vi "2_AdvancedDemo_TH260Histo.vi"() -> ()   [LabVIEW 2017]
uses:
  Types/TH260_InputChannel.ctl
  Types/TH260_UIThread_Cmds.ctl
  Types/TH260_UIThread_Data.ctl
  _lib/PQ/TimeHarp260/TH260_InitInfo.ctl
  _lib/PQ/TimeHarp260/TH260_MeasMode.ctl
  _lib/PQ/TimeHarp260/TH260_TimingMode.ctl
  <vilib>/Utility/error.llb/DialogType.ctl
  _lib/PQ/TimeHarp260/th260lib_x86_x64_UIThread.llb/TH260_DllPath_global.vi
  <vilib>/Utility/error.llb/Error Cluster From Error Code.vi
  _lib/PQ/TimeHarp260/TH260_LibVersion_global.vi
  <vilib>/ErrorRing/Error Ring.xnode
panel:
  in  "Settings":bool=TRUE
  in  "Run continuously":bool=TRUE caption="Conti."
  in  "Start":bool
  in  "Scale":bool
  out "CountRates":i32[](graph)
  in  "HistoLength":i32(ring)=6 caption="Num Bins" items=["1024", "2048", "4096", "8192", "16384", "32768"]
  in  "OvlLevel":u32=100000 caption="Ovl.Level" min=1 step=1
  in  "StopOvl.":bool=TRUE
  in  "AcqTime":i32=1000 caption="Acqu.     ms" min=1 max=360000000 step=1
  in  "Binning":i32(ring) caption="Resol.      ps" items=["25", "50", "100", "200", "400", "800", "1600", "3200", "6400", "12800", "25600", "51200", "102400", "204800", "409600", "819200", "1638400", "3276800", "6553600", "13107200", "26214400", "52428800"]
  in  "HistoOffset":i32 caption="Offset      ns" min=0 max=100000000 step=1
  out "HistoGraph":T1(graph)={0.0, "Resolution"=0.001, "Histogram"=array8x1024[8192 elements]}
  in  "SyncTrgEdge":i32(ring) caption="Edge" items=["falling", "rising"]
  in  "SyncTrgLevel":i32=-100 caption="Level        mV" min=-1200 max=1200 step=1
  in  "SyncCFDLevel":i32=-100 caption="Level        mV" min=-1200 max=0 step=1
  in  "SyncZeroX":i32=-10 caption="ZeroCr.    mV" min=-40 max=0 step=1
  in  "SyncDivider":i32(ring)=3 caption="Divider" items=["1", "2", "4", "8"]
  in  "SyncOffset":i32 caption="Offset        ps" min=-99999 max=99999 step=1
  in  "Channels":T2[](array[typedef])=[{"Name"="Inp.Chan 1", "Enable"=TRUE, "Offset"=0, "CFDLevel"=50, "ZeroX"=10, "dtcode"=0, "TrgLevel"=-100, "TrgEdge"=0}, {"Name"="Inp.Chan 2", "Enable"=TRUE, "Offset"=0, "CFDLevel"=50, "ZeroX"=10, "dtcode"=0, "TrgLevel"=-100, "TrgEdge"=0}, {"Name"="Inp.Chan 3", "Enable"=TRUE, "Offset"=0, "CFDLevel"=50, "ZeroX"=10, "dtcode"=0, "TrgLevel"=-100, "TrgEdge"=0}, {"Name"="Inp.Chan 4", "Enable"=TRUE, "Offset"=0, "CFDLevel"=50, "ZeroX"=10, "dtcode"=0, "TrgLevel"=-100, "TrgEdge"=0}, {"Name"="Inp.Chan 5", "Enable"=TRUE, "Offset"=0, "CFDLevel"=50, "ZeroX"=10, "dtcode"=0, "TrgLevel"=-100, "TrgEdge"=0}, {"Name"="Inp.Chan 6", "Enable"=TRUE, "Offset"=0, "CFDLevel"=50, "ZeroX"=10, "dtcode"=0, "TrgLevel"=-100, "TrgEdge"=0}, {"Name"="Inp.Chan 7", "Enable"=TRUE, "Offset"=0, "CFDLevel"=50, "ZeroX"=10, "dtcode"=0, "TrgLevel"=-100, "TrgEdge"=0}, {"Name"="Inp.Chan 8", "Enable"=TRUE, "Offset"=0, "CFDLevel"=50, "ZeroX"=10, "dtcode"=0, "TrgLevel"=-100, "TrgEdge"=0}] {"TrgEdge" items=["falling", "rising"]; "TrgLevel" min=-1200 max=1200 step=1; "dtcode" items=["24", "44", "66", "88", "112", "135", "160", "180"]; "ZeroX" min=-40 max=0 step=1; "Offset" min=-99999 max=99999 step=1; "CFDLevel" min=-1200 max=0 step=1}
  out "SyncRate":string="Sync Rate: 0 cps\n"
  out "OverFlow":bool caption="Overflow:"
  out "Status":string="Initialized!"
  # "Histogram"
  # "Sync"
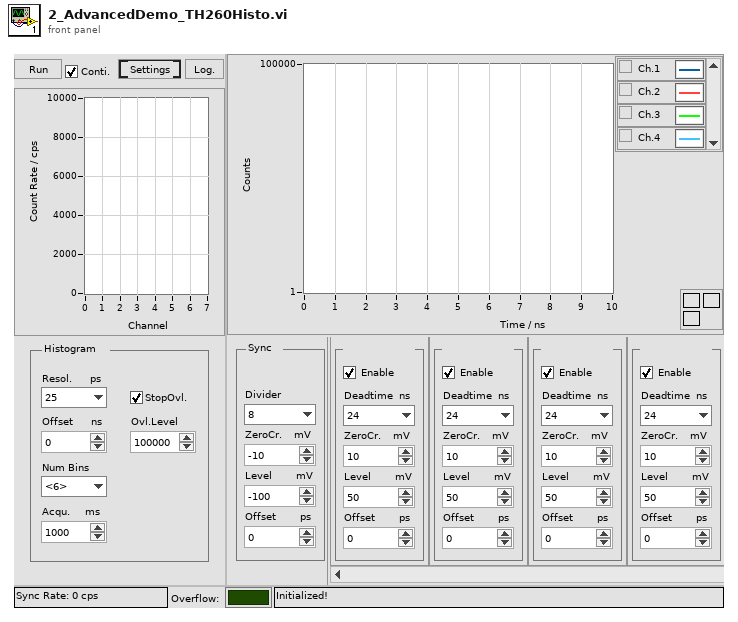
[diagram p1: front panel]
types:
  T1 = cluster{dbl, "Resolution":dbl, "Histogram":u32[][]}
  T2 = typedef "TH260_InputChannel.ctl" = cluster{"Name":string, "Enable":bool, "Offset":i32, "CFDLevel":i32, "ZeroX":i32, "dtcode":i32, "TrgLevel":i32, "TrgEdge":i32}
  T3 = typedef "TH260_UIThread_Data.ctl" = cluster{"Init Info":T4, "DevIdx":i32, "Channels":T2[], "CurrentChannels":i32[], "AcqTime":i32, "Binning":i32, "HistoOffset":i32, "HistoLen":i32, "StopOvl.":bool, "OvlLevel":u32, "StartMeas":bool, "HistoLength":i32, "Resolution":dbl, "Run cont.":bool, "Status":string, "SyncRate":i32, "BitShift":i32, "HistoAcqTime":dbl, "SyncTrgEdge":i32, "SyncTrgLevel":i32, "SyncCFDLevel":i32, "SyncZeroX":i32, "SyncDivider":i32, "SyncOffset":i32}
  T4 = typedef "TH260_InitInfo.ctl" = cluster{"Library Version":string, "Serial No.":string, "Model":string, "Partnum":string, "Version":string, "features":i32, "nchannels":i32, "Base Resolution":dbl, "Bin Steps":i32}
  T5 = typedef "TH260_UIThread_Cmds.ctl" = enum16{"Idle", "Init", "SetInpChanEnable", "SetInpChanOffset", "SetInpChanCFD", "SetInpChanTrg", "SetInpChanDeadtime", "SetSyncDivider", "SetSyncCFD", "SetSyncTrg", "SetSyncOffset", "SetBinning", "SetHistoOffset", "SetHistoLen", "SetStopOvl", "SetBitShift", "SetHistoAcqTime", "GetRates", "StartMeas", "StopMeas", "AbortMeas", "GetResolution", "GetHisto", "ReadFiFo", "WriteStatus", "Resize", "EnableControls", "DisableControls", "Error", "Exit"}
  T6 = enum8{"Enabled", "Disabled", "Disabled and Grayed Out"}
  T7 = typedef "TH260_TimingMode.ctl" = i32
  T8 = typedef "TH260_MeasMode.ctl" = i32
  T9 = typedef "DialogType.ctl" = u16
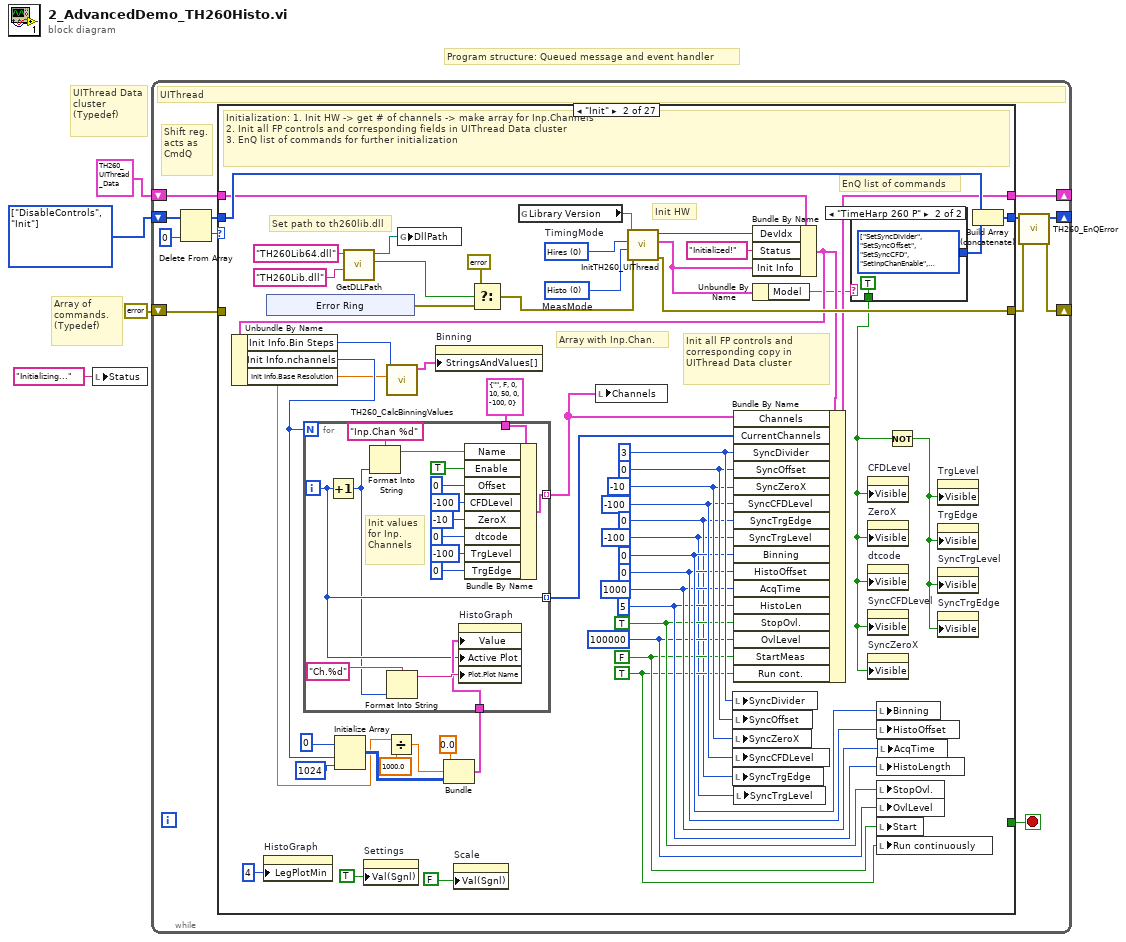
[diagram p0: block diagram]
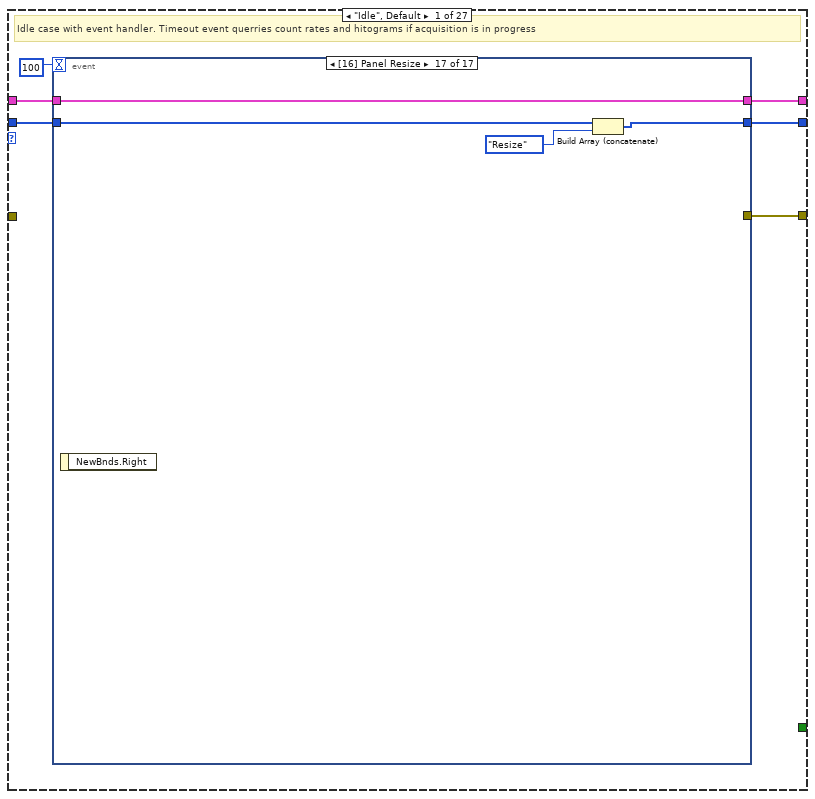
[diagram p2: hidden frame]
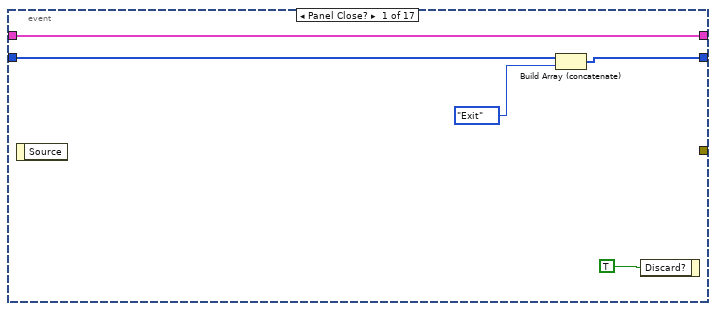
[diagram p3: hidden frame]
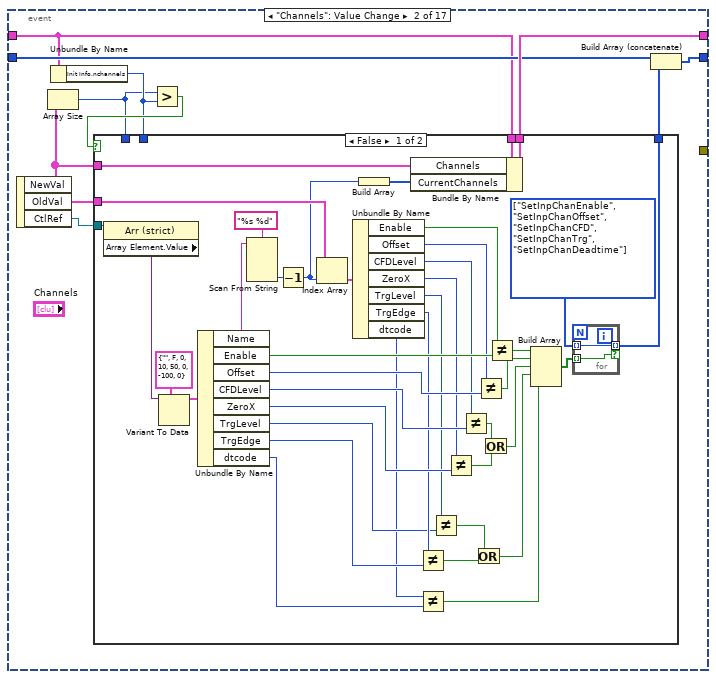
[diagram p4: hidden frame]
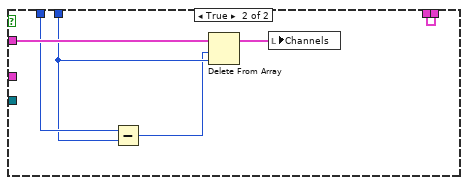
[diagram p5: hidden frame]
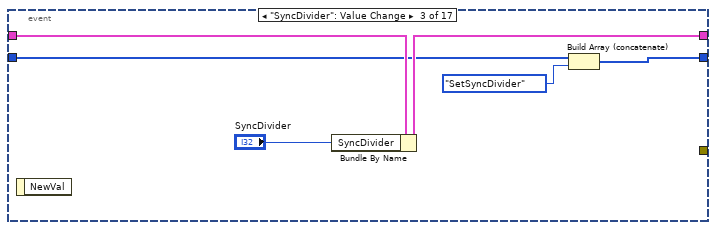
[diagram p6: hidden frame]
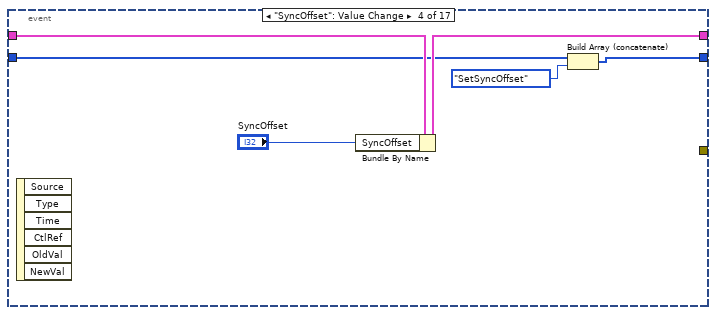
[diagram p7: hidden frame]
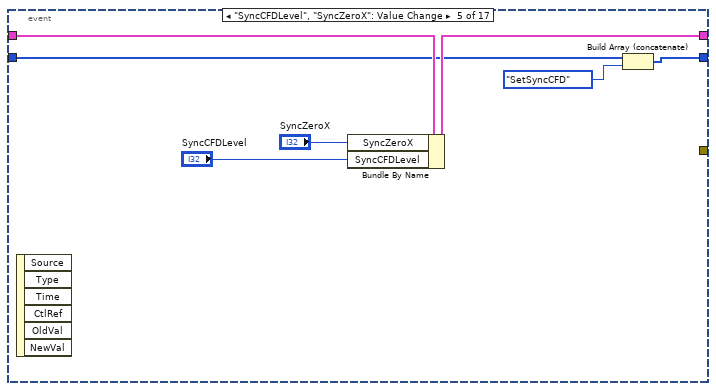
[diagram p8: hidden frame]
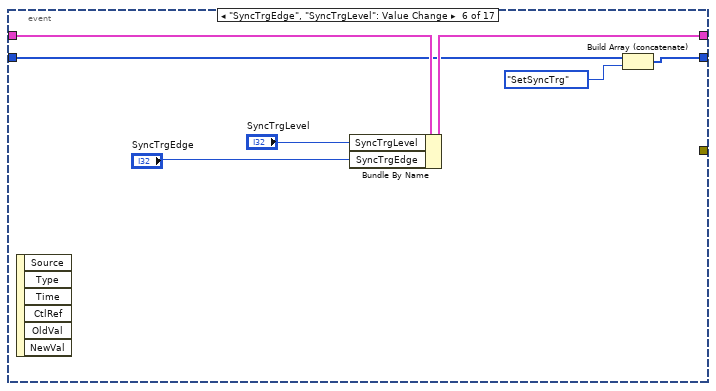
[diagram p9: hidden frame]
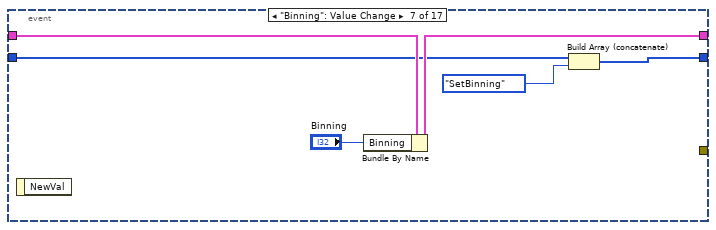
[diagram p10: hidden frame]
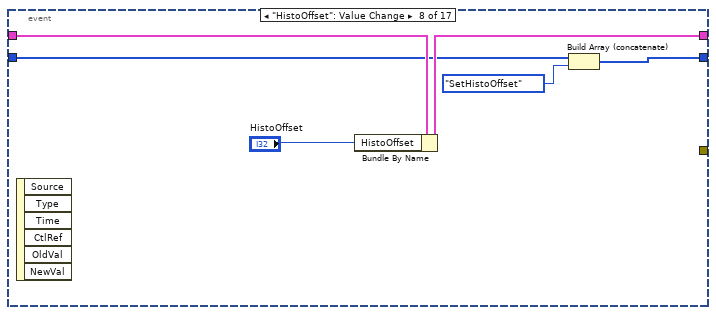
[diagram p11: hidden frame]
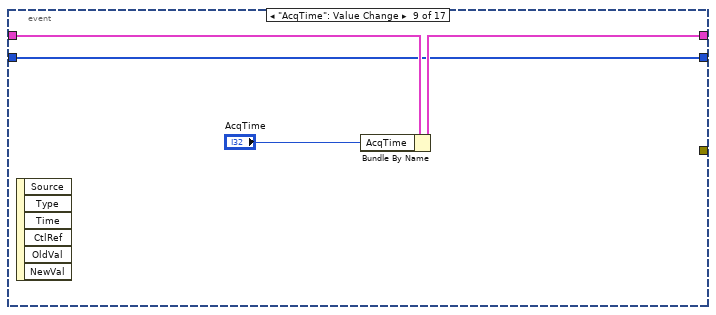
[diagram p12: hidden frame]
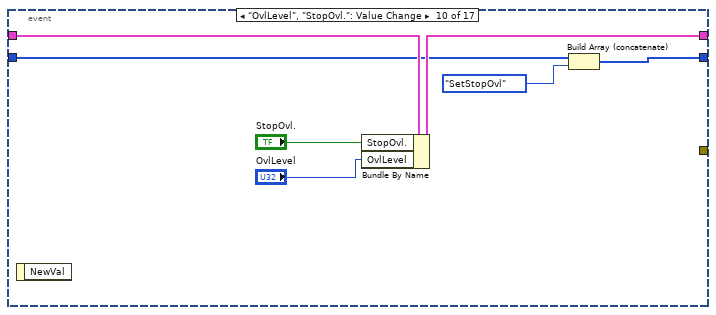
[diagram p13: hidden frame]
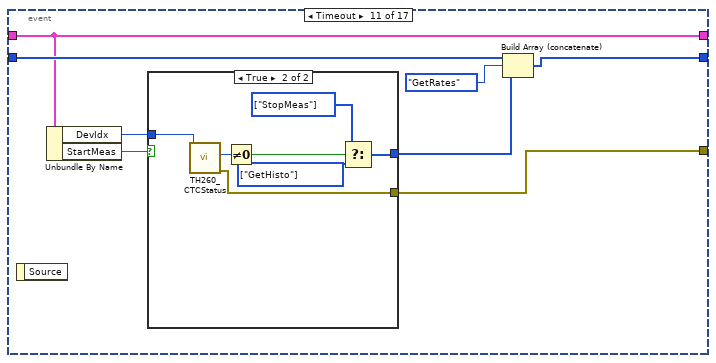
[diagram p14: hidden frame]
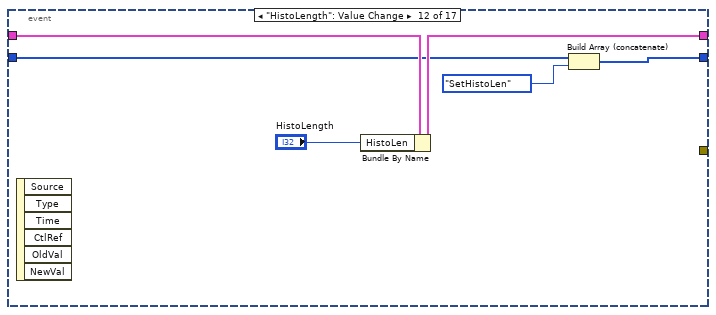
[diagram p16: hidden frame]
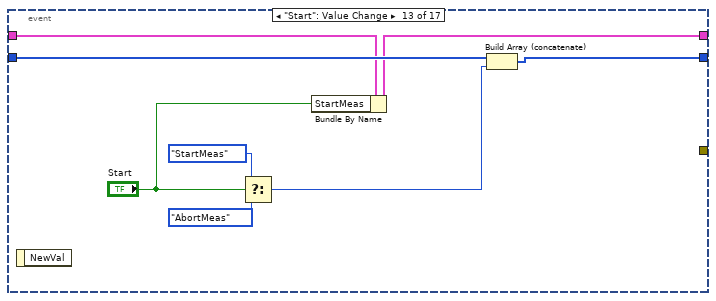
[diagram p17: hidden frame]
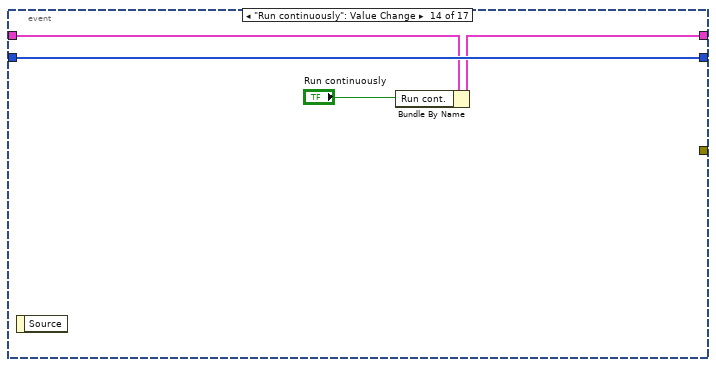
[diagram p18: hidden frame]
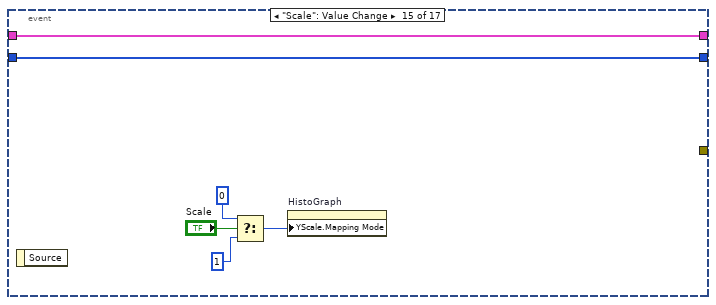
[diagram p19: hidden frame]
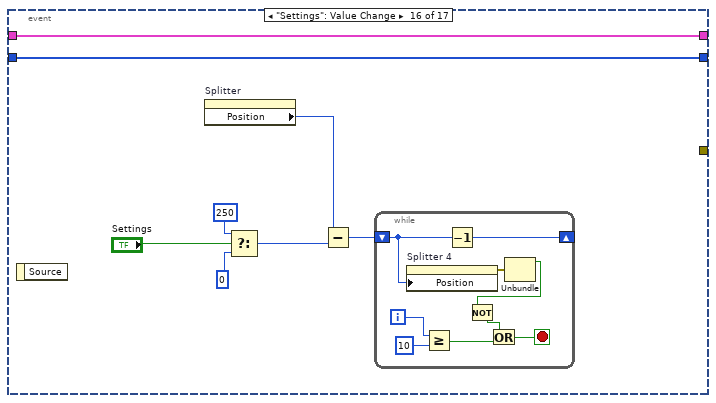
[diagram p20: hidden frame]
diagram:
  w3 = T5[] [enum."DisableControls", enum."Init"] items=["Idle", "Init", "SetInpChanEnable", "SetInpChanOffset", "SetInpChanCFD", "SetInpChanTrg", "SetInpChanDeadtime", "SetSyncDivider", "SetSyncCFD", "SetSyncTrg", "SetSyncOffset", "SetBinning", "SetHistoOffset", "SetHistoLen", "SetStopOvl", "SetBitShift", "SetHistoAcqTime", "GetRates", "StartMeas", "StopMeas", "AbortMeas", "GetResolution", "GetHisto", "ReadFiFo", "WriteStatus", "Resize", "EnableControls", "DisableControls", "Error", "Exit"]
  # "Array of commands.\n(Typedef)"
  # "Program structure: Queued message and event handler"
  # "UIThread Data cluster\n(Typedef)"
  n1 = local write "Status"("Initializing..." ("Status")) -> ()
  n2 = while {
    shift-right: [w5] -> _
    shift-left: w3 -> [w12]
    shift-right: [w15] -> _
    shift-left: T3 {"Init Info"={"Library Version"="", "Serial No."="", "Model"="", "Partnum"="", "Version"="", "features"=0, "nchannels"=0, "Base Resolution"=0.0, "Bin Steps"=0}, "DevIdx"=0, "Channels"=[], "CurrentChannels"=[], "AcqTime"=1, "Binning"=1, "HistoOffset"=1, "HistoLen"=1024, "StopOvl."=FALSE, "OvlLevel"=1024, "StartMeas"=FALSE, "HistoLength"=0, "Resolution"=0.0, "Run cont."=FALSE, "Status"="", "SyncRate"=0, "BitShift"=0, "HistoAcqTime"=0.0, "SyncTrgEdge"=0, "SyncTrgLevel"=-100, "SyncCFDLevel"=10, "SyncZeroX"=3, "SyncDivider"=3, "SyncOffset"=0} -> [w14]
    shift-right: [w7] -> _
    shift-left: errorcluster {"status"=FALSE, "code"=0, "source"=""} ("error IO") -> [w13]
    stop <- w16 stop-if-true
    # "Shift reg.\nacts as\nCmdQ"
    # "UIThread"
    n3 = Delete From Array(array=w12, index=0) -> (deleted portion=w10:T5, array with subset deleted=w9:T5[])  [unwired: 1 in]
    n4 = case shown="\"Init\"" w10 {
      tunnel: [w22 w245 w278 w292 w306 w321 w336 w352 w361 w367 w369 w376 w384 w392 w397 w409 w424 w432 w446 w460 w487 w512 w525 w532 w544 w550 w554] -> w6
      tunnel: [_ _ _ _ _ _ _ _ _ _ _ _ _ _ _ _ _ _ _ _ _ _ _ _ _ _ TRUE] -> w16
      tunnel: [w21 w225 w281 w295 w309 w324 w339 w354 w362 w368 w373 w380 w385 w387 w398 w408 w430 w435 w449 w456 w486 w511 w513 w531 w543 w551 w557] -> w15
      tunnel: w14 -> [w20 w230 w281 w295 w309 w324 w339 w354 w362 w368 w373 w380 w385 w388 w398 w408 w430 w436 w450 w457 w486 w511 w513 w531 w543 w551 w557]
      tunnel: [w17 w247 w279 w293 w307 w322 w337 w350 w360 w366 w372 w379 w383 w391 w396 w407 w429 w438 w452 w458 w482 _ _ _ _ _ w555] -> w8
      tunnel: w13 -> [_ _ _ _ _ _ _ _ _ _ _ _ _ _ _ _ _ _ _ _ _ _ _ _ _ w552 _]
      tunnel: w9 -> [w19 w246 w278 w292 w306 w321 w336 w352 w361 w367 w369 w375 w384 w392 w397 w409 w425 w433 w447 w460 w487 w512 w525 w532 w544 _ w554]
      frame "Idle", Default {
        # "Idle case with event handler. Timeout event querries count rates and hitograms if acquisition is in progress"
        n5 = event shown="[16] Panel Resize" {
          selector: _ -> [_ _ _ _ _ _ _ _ _ _ _ _ _ _ _ _ _]
          dyn-events: _ -> [_ _ _ _ _ _ _ _ _ _ _ _ _ _ _ _ _]
          timeout: 100 -> [_ _ _ _ _ _ _ _ _ _ _ _ _ _ _ _ _]
          tunnel: [w23 w33 w88 w94 w101 w108 w114 w120 w125 w131 w141 w152 w160 w168 w174 w182 w192] -> w22
          tunnel: [w26 w36 w91 w97 w104 w111 w117 w123 w127 w134 w140 w155 w158 w166 w173 w181 w195] -> w21
          tunnel: w20 -> [w26 w32 w92 w98 w105 w112 w118 w124 w128 w135 w140 w156 w159 w167 w173 w181 w195]
          tunnel: w19 -> [w25 w35 w90 w96 w103 w110 w116 w122 w125 w133 w143 w154 w162 w168 w174 w182 w193]
          tunnel: [_ _ _ _ _ _ _ _ _ _ w136 _ _ _ _ _ _] -> w17
          event Panel Close? {
            n6 = event-data() -> ()  [unwired: 1 in, 1 out]
            n7 = Build Array (concatenate)(w25, TH260_UIThread_Cmds."Exit") -> (w23:T5[])
            n8 = event-data("Discard?"=TRUE) -> ()  [unwired: 1 in, 1 out]
          }
          event "Channels": Value Change {
            n9 = event-data() -> ("NewVal"=w31:T2[], "OldVal"=w37:T2[], "CtlRef"=w38:refnum<vi>)  [unwired: 1 in]
            n10 = Array Size(array=w31) -> (size(s)=w28:i32)
            n11 = Unbundle By Name(w32) -> ("Init Info.nchannels"=w29:i32)
            n12 = Greater?(x=w28, y=w29) -> (0:w30:bool)
            n13 = case shown="False" w30 {
              tunnel: w38 -> [w78 _]
              tunnel: w37 -> [w72 _]
              tunnel: [w55 w86] -> w36
              tunnel: [w53 _] -> w34
              tunnel: w32 -> [w50 w86]
              tunnel: w31 -> [w49 w85]
              tunnel: w29 -> [_ w83]
              tunnel: w28 -> [_ w84]
              frame False {
                w56 = T5[] [enum."SetInpChanEnable", enum."SetInpChanOffset", enum."SetInpChanCFD", enum."SetInpChanTrg", enum."SetInpChanDeadtime"] items=["Idle", "Init", "SetInpChanEnable", "SetInpChanOffset", "SetInpChanCFD", "SetInpChanTrg", "SetInpChanDeadtime", "SetSyncDivider", "SetSyncCFD", "SetSyncTrg", "SetSyncOffset", "SetBinning", "SetHistoOffset", "SetHistoLen", "SetStopOvl", "SetBitShift", "SetHistoAcqTime", "GetRates", "StartMeas", "StopMeas", "AbortMeas", "GetResolution", "GetHisto", "ReadFiFo", "WriteStatus", "Resize", "EnableControls", "DisableControls", "Error", "Exit"]
                n14 = property class="Arr (strict)"(reference=w78) -> ("Array Element.Value"=w77:variant)  [unwired: 1 in, 2 out]
                n15 = Variant To Data(type=T2 {"Name"="", "Enable"=FALSE, "Offset"=0, "CFDLevel"=10, "ZeroX"=50, "dtcode"=0, "TrgLevel"=-100, "TrgEdge"=0} ("Channel"), Variant=w77) -> (data=w54:T2)  [unwired: 1 in, 1 out]
                n16 = Unbundle By Name(w54) -> ("Name"=w75:string, "Enable"=w69:bool, "Offset"=w67:i32, "CFDLevel"=w65:i32, "ZeroX"=w63:i32, "TrgLevel"=w46:i32, "TrgEdge"=w45:i32, "dtcode"=w40:i32)
                n17 = Scan From String(format string="%s %d", input string=w75) -> (output 2=w73:i32)  [unwired: 5 in, 3 out]
                n18 = Decrement(x=w73) -> (x-1=w52:i32)
                n19 = Index Array(array=w72, index=w52) -> (element=w71:T2)
                n20 = Unbundle By Name(w71) -> ("Enable"=w70:bool, "Offset"=w68:i32, "CFDLevel"=w66:i32, "ZeroX"=w64:i32, "TrgLevel"=w48:i32, "TrgEdge"=w47:i32, "dtcode"=w41:i32)
                n21 = Build Array(w52) -> (w51:i32[])
                n22 = Bundle By Name(cluster=w50, "Channels"=w49, "CurrentChannels"=w51) -> (w55:T3)
                n23 = Not Equal?(x=w47, y=w45) -> (x != y?=w43:bool)
                n24 = Not Equal?(x=w41, y=w40) -> (x != y?=w39:bool)
                n25 = Not Equal?(x=w48, y=w46) -> (x != y?=w44:bool)
                n26 = Not Equal?(x=w64, y=w63) -> (x != y?=w58:bool)
                n27 = Not Equal?(x=w66, y=w65) -> (x != y?=w59:bool)
                n28 = Or(x=w44, y=w43) -> (x .or. y?=w42:bool)
                n29 = Not Equal?(x=w68, y=w67) -> (x != y?=w61:bool)
                n30 = Or(x=w59, y=w58) -> (x .or. y?=w57:bool)
                n31 = Not Equal?(x=w70, y=w69) -> (x != y?=w62:bool)
                n32 = Build Array(w62, w61, w57, w42, w39) -> (w60:bool[])
                n33 = for {
                  tunnel: w60 -> [w79] mode=indexing
                  tunnel: w56 -> [w80] mode=indexing
                  tunnel: [w80] -> w53 mode=indexing if=w79
                }
              }
              frame True {
                n34 = Subtract(x=w84, y=w83) -> (x-y=w82:i32)
                n35 = Delete From Array(array=w85, length=w82, index=w83) -> (array with subset deleted=w81:T2[])  [unwired: 1 out]
                n36 = local write "Channels"(w81) -> ()
              }
            }
            n37 = Build Array (concatenate)(w35, w34) -> (w33:T5[])
          }
          event "SyncDivider": Value Change {
            n38 = event-data() -> ()  [unwired: 1 in, 1 out]
            n39 = Bundle By Name(cluster=w92, "SyncDivider"="SyncDivider") -> (w91:T3)
            n40 = Build Array (concatenate)(w90, TH260_UIThread_Cmds."SetSyncDivider") -> (w88:T5[])
          }
          event "SyncOffset": Value Change {
            n41 = event-data() -> ()  [unwired: 1 in, 6 out]
            n42 = Bundle By Name(cluster=w98, "SyncOffset"="SyncOffset") -> (w97:T3)
            n43 = Build Array (concatenate)(w96, TH260_UIThread_Cmds."SetSyncOffset") -> (w94:T5[])
          }
          event "SyncCFDLevel", "SyncZeroX": Value Change {
            n44 = event-data() -> ()  [unwired: 1 in, 6 out]
            n45 = Bundle By Name(cluster=w105, "SyncZeroX"="SyncZeroX", "SyncCFDLevel"="SyncCFDLevel") -> (w104:T3)
            n46 = Build Array (concatenate)(w103, TH260_UIThread_Cmds."SetSyncCFD") -> (w101:T5[])
          }
          event "SyncTrgEdge", "SyncTrgLevel": Value Change {
            n47 = event-data() -> ()  [unwired: 1 in, 6 out]
            n48 = Bundle By Name(cluster=w112, "SyncTrgLevel"="SyncTrgLevel", "SyncTrgEdge"="SyncTrgEdge") -> (w111:T3)
            n49 = Build Array (concatenate)(w110, TH260_UIThread_Cmds."SetSyncTrg") -> (w108:T5[])
          }
          event "Binning": Value Change {
            n50 = event-data() -> ()  [unwired: 1 in, 1 out]
            n51 = Bundle By Name(cluster=w118, "Binning"="Binning") -> (w117:T3)
            n52 = Build Array (concatenate)(w116, TH260_UIThread_Cmds."SetBinning") -> (w114:T5[])
          }
          event "HistoOffset": Value Change {
            n53 = event-data() -> ()  [unwired: 1 in, 6 out]
            n54 = Bundle By Name(cluster=w124, "HistoOffset"="HistoOffset") -> (w123:T3)
            n55 = Build Array (concatenate)(w122, TH260_UIThread_Cmds."SetHistoOffset") -> (w120:T5[])
          }
          event "AcqTime": Value Change {
            n56 = event-data() -> ()  [unwired: 1 in, 6 out]
            n57 = Bundle By Name(cluster=w128, "AcqTime"="AcqTime") -> (w127:T3)
          }
          event "OvlLevel", "StopOvl.": Value Change {
            n58 = event-data() -> ()  [unwired: 1 in, 1 out]
            n59 = Bundle By Name(cluster=w135, "StopOvl."="StopOvl.", "OvlLevel"="OvlLevel") -> (w134:T3)
            n60 = Build Array (concatenate)(w133, TH260_UIThread_Cmds."SetStopOvl") -> (w131:T5[])
          }
          event Timeout {
            n61 = event-data() -> ()  [unwired: 1 in, 1 out]
            n62 = Unbundle By Name(w140) -> ("DevIdx"=w138:i32, "StartMeas"=w139:bool)
            n63 = case shown="True" w139 {
              tunnel: w138 -> [_ w150]
              tunnel: [_ w148] -> w137
              tunnel: [_ w145] -> w136
              frame False {
              }
              frame True {
                w146 = T5[] [enum."GetHisto"] items=["Idle", "Init", "SetInpChanEnable", "SetInpChanOffset", "SetInpChanCFD", "SetInpChanTrg", "SetInpChanDeadtime", "SetSyncDivider", "SetSyncCFD", "SetSyncTrg", "SetSyncOffset", "SetBinning", "SetHistoOffset", "SetHistoLen", "SetStopOvl", "SetBitShift", "SetHistoAcqTime", "GetRates", "StartMeas", "StopMeas", "AbortMeas", "GetResolution", "GetHisto", "ReadFiFo", "WriteStatus", "Resize", "EnableControls", "DisableControls", "Error", "Exit"]
                w147 = T5[] [enum."StopMeas"] items=["Idle", "Init", "SetInpChanEnable", "SetInpChanOffset", "SetInpChanCFD", "SetInpChanTrg", "SetInpChanDeadtime", "SetSyncDivider", "SetSyncCFD", "SetSyncTrg", "SetSyncOffset", "SetBinning", "SetHistoOffset", "SetHistoLen", "SetStopOvl", "SetBitShift", "SetHistoAcqTime", "GetRates", "StartMeas", "StopMeas", "AbortMeas", "GetResolution", "GetHisto", "ReadFiFo", "WriteStatus", "Resize", "EnableControls", "DisableControls", "Error", "Exit"]
                n64 = call "TH260_CTCStatus.vi"("devidx"=w150) -> ("error out"=w145:errorcluster, "ctcstatus"=w149:i32)  [unwired: 8 in, 1 out]
                n65 = Not Equal To 0?(x=w149) -> (x != 0?=w144:bool)
                n66 = Select(t=w147, s=w144, f=w146) -> (s? t:f=w148:T5[])
              }
            }
            n67 = Build Array (concatenate)(w143, TH260_UIThread_Cmds."GetRates", w137) -> (w141:T5[])
          }
          event "HistoLength": Value Change {
            n68 = event-data() -> ()  [unwired: 1 in, 6 out]
            n69 = Bundle By Name(cluster=w156, "HistoLen"="HistoLength") -> (w155:T3)
            n70 = Build Array (concatenate)(w154, TH260_UIThread_Cmds."SetHistoLen") -> (w152:T5[])
          }
          event "Start": Value Change {
            n71 = event-data() -> ()  [unwired: 1 in, 1 out]
            n72 = Select(t=TH260_UIThread_Cmds."StartMeas", s="Start", f=TH260_UIThread_Cmds."AbortMeas") -> (s? t:f=w161:T5)
            n73 = Bundle By Name(cluster=w159, "StartMeas"="Start") -> (w158:T3)
            n74 = Build Array (concatenate)(w162, w161) -> (w160:T5[])
          }
          event "Run continuously": Value Change {
            n75 = event-data() -> ()  [unwired: 1 in, 1 out]
            n76 = Bundle By Name(cluster=w167, "Run cont."="Run continuously") -> (w166:T3)
          }
          event "Scale": Value Change {
            n77 = event-data() -> ()  [unwired: 1 in, 1 out]
            n78 = Select(t=u8 0 ("Y Scale.Mapping Mode"), s="Scale", f=u8 1 ("Y Scale.Mapping Mode")) -> (s? t:f=w169:u8)
            n79 = property on="HistoGraph" class="WFGraph (strict)"("YScale.Mapping Mode"=w169) -> ()  [unwired: 2 in, 2 out]
          }
          event "Settings": Value Change {
            n80 = event-data() -> ()  [unwired: 1 in, 1 out]
            n81 = property on="Splitter" class="Splitter"() -> ("Position"=w180:i32)  [unwired: 2 in, 2 out]
            n82 = Select(t=250 ("PosT"), s="Settings", f=0 ("PosF")) -> (s? t:f=w177:i32)
            n83 = Subtract(x=w180, y=w177) -> (x-y=w176:i32)
            n84 = while {
              shift-right: [w191] -> _
              shift-left: w176 -> [w184]
              i -> [w190]
              stop <- w187 stop-if-true
              n85 = property on="Splitter 4" class="Splitter"("Position"=w184) -> (error out=w183:errorcluster)  [unwired: 2 in, 1 out]
              n86 = Greater Or Equal?(x=w190, y=10) -> (x >= y?=w188:bool)
              n87 = Decrement(x=w184) -> (x-1=w191:i32)
              n88 = Unbundle(w183) -> ("status"=w186:bool)  [unwired: 2 out]
              n89 = Not(x=w186) -> (.not. x?=w185:bool)
              n90 = Or(x=w185, y=w188) -> (x .or. y?=w187:bool)
            }
          }
          event Panel Resize {
            n91 = event-data() -> ()  [unwired: 1 in, 1 out]
            n92 = Build Array (concatenate)(w193, TH260_UIThread_Cmds."Resize") -> (w192:T5[])
          }
        }
      }
      frame "Init" {
        w198 = -100 ("SyncTrgLevel")
        w199 = 0 ("SyncTrgEdge")
        w204 = T7 0 items=["Hires", "Lowres"]  # TimingMode
        w205 = T8 0 items=["Histo"=0, "T2"=2, "T3"=3]  # MeasMode
        w232 = TRUE ("Run cont.")
        w234 = FALSE ("StartMeas")
        w235 = u32 100000 ("OvlLevel")
        w236 = TRUE ("StopOvl.")
        w237 = 5 ("HistoLen")
        w238 = 1000 ("AcqTime")
        w239 = 0 ("HistoOffset")
        w240 = 0 ("Binning")
        w241 = -100 ("SyncLevel")
        w242 = -10 ("SyncZeroX")
        w243 = 0 ("SyncOffset")
        w244 = 3 ("SyncDivider")
        # "Init HW"
        # "Set path to th260lib.dll"
        # "Init all FP controls and corresponding copy in UIThread Data cluster"
        # "EnQ list of commands"
        # "Array with Inp.Chan."
        # "Initialization: 1. Init HW -> get # of channels -> make array for Inp.Channels\n2. Init all FP controls and corresponding fields in UIThread Data cluster\n3. EnQ list of commands for further initialization"
        n93 = property on="HistoGraph" class="WFGraph (strict)"("LegPlotMin"=u32 4 ("Legend:Plot Minimum")) -> ()  [unwired: 2 in, 2 out]
        n94 = xnode "Error Ring"() -> ("error out"=w218:errorcluster)
        n95 = call "GetDLLPath.vi"("DllName_32bit"="TH260Lib.dll" ("name or relative path"), "DllName_64bit"="TH260Lib64.dll" ("name or relative path")) -> ("file exists?"=w220:bool, "DLLPath"=w221:path)  [unwired: 8 in]
        n96 = property on="Settings" class="Bool (strict)"("Val(Sgnl)"=TRUE ("Value (Signaling)")) -> ()  [unwired: 2 in, 2 out]
        n97 = global write "TH260_DllPath_global.vi" "DllPath"(w221) -> ()
        n98 = property on="Scale" class="Bool (strict)"("Val(Sgnl)"=FALSE ("Value (Signaling)")) -> ()  [unwired: 2 in, 2 out]
        n99 = Select(t=errorcluster {"status"=FALSE, "code"=0, "source"=""} ("error IO"), s=w220, f=w218) -> (s? t:f=w226:errorcluster)
        n100 = global read "TH260_LibVersion_global.vi" "Library Version"() -> (w217:string)
        n101 = call "InitTH260_UIThread.vi"("error in (no error)"=w226, "MeasMode"=w205, "TimingMode"=w204, "Library Version"=w217) -> ("error out"=w247:errorcluster, "Init Info"=w203:T4, "DevIdx"=w249:i32)  [unwired: 5 in]
        n102 = local write "SyncDivider"(w244) -> ()
        n103 = local write "SyncOffset"(w243) -> ()
        n104 = local write "SyncZeroX"(w242) -> ()
        n105 = local write "SyncCFDLevel"(w241) -> ()
        n106 = local write "SyncTrgEdge"(w199) -> ()
        n107 = local write "SyncTrgLevel"(w198) -> ()
        n108 = Bundle By Name(cluster=w230, "DevIdx"=w249, "Status"="Initialized!", "Init Info"=w203) -> (w229:T3)
        n109 = Unbundle By Name(w229) -> ("Init Info.Bin Steps"=w228:i32, "Init Info.nchannels"=w207:i32, "Init Info.Base Resolution"=w197:dbl)
        n110 = Initialize Array(u32 0, w207, 1024 ("dimension size")) -> (w211:u32[][])
        n111 = Divide(x=w197, y=1000.0) -> (x/y=w212:dbl)
        n112 = call "TH260_CalcBinningValues.vi"("BaseRes"=w197, "Bin Steps"=w228) -> ("BinningValues"=w233:cluster{"String":string, "Value":i32}[])  [unwired: 9 in]
        n113 = property on="Binning" class="Ring (strict)"("StringsAndValues[]"=w233) -> ()  [unwired: 2 in, 2 out]
        n114 = Bundle(0.0, w212, w211) -> (w210:cluster{dbl, dbl, u32[][]})  [unwired: 1 in]
        n115 = for {
          N: w207 -> [_]
          tunnel: T2 {"Name"="", "Enable"=FALSE, "Offset"=0, "CFDLevel"=10, "ZeroX"=50, "dtcode"=0, "TrgLevel"=-100, "TrgEdge"=0} ("Channel") -> [w274]
          tunnel: [w273] -> w206 mode=indexing
          tunnel: [w263] -> w208 mode=indexing
          tunnel: w210 -> [w264]
          i -> [w263]
          # "Init values for Inp. Channels"
          n116 = Increment(x=w263) -> (x+1=w262:i32)
          n117 = Format Into String(format string="Inp.Chan %d", w262) -> (resulting string=w271:string)  [unwired: 2 in, 1 out]
          n118 = Format Into String(format string="Ch.%d", w262) -> (resulting string=w265:string)  [unwired: 2 in, 1 out]
          n119 = property on="HistoGraph" class="WFGraph (strict)"("Value"=w264, "Active Plot"=w263, "Plot.Plot Name"=w265) -> ()  [unwired: 2 in, 2 out]
          n120 = Bundle By Name(cluster=w274, "Name"=w271, "Enable"=TRUE, "Offset"=0, "CFDLevel"=-100 ("CFDZeroX"), "ZeroX"=-10 ("CFDLevel"), "dtcode"=0, "TrgLevel"=-100, "TrgEdge"=0) -> (w273:T2)
        }
        n121 = local write "Channels"(w206) -> ()
        n122 = Bundle By Name(cluster=w229, "Channels"=w206, "CurrentChannels"=w208, "SyncDivider"=w244, "SyncOffset"=w243, "SyncZeroX"=w242, "SyncCFDLevel"=w241, "SyncTrgEdge"=w199, "SyncTrgLevel"=w198, "Binning"=w240, "HistoOffset"=w239, "AcqTime"=w238, "HistoLen"=w237, "StopOvl."=w236, "OvlLevel"=w235, "StartMeas"=w234, "Run cont."=w232) -> (w225:T3)
        n123 = Unbundle By Name(w203) -> ("Model"=w202:string)
        n124 = case shown="\"TimeHarp 260 P\"" w202 {
          tunnel: [FALSE TRUE] -> w201
          tunnel: [w250 w252] -> w196
          frame Default {
            w250 = T5[] [enum."SetSyncDivider", enum."SetSyncOffset", enum."SetSyncTrg", enum."SetInpChanEnable", enum."SetInpChanOffset", enum."SetInpChanTrg", enum."SetBinning", enum."SetHistoOffset", enum."SetHistoLen", enum."SetStopOvl", enum."Resize", enum."EnableControls", enum."WriteStatus"] items=["Idle", "Init", "SetInpChanEnable", "SetInpChanOffset", "SetInpChanCFD", "SetInpChanTrg", "SetInpChanDeadtime", "SetSyncDivider", "SetSyncCFD", "SetSyncTrg", "SetSyncOffset", "SetBinning", "SetHistoOffset", "SetHistoLen", "SetStopOvl", "SetBitShift", "SetHistoAcqTime", "GetRates", "StartMeas", "StopMeas", "AbortMeas", "GetResolution", "GetHisto", "ReadFiFo", "WriteStatus", "Resize", "EnableControls", "DisableControls", "Error", "Exit"]
          }
          frame "TimeHarp 260 P" {
            w252 = T5[] [enum."SetSyncDivider", enum."SetSyncOffset", enum."SetSyncCFD", enum."SetInpChanEnable", enum."SetInpChanOffset", enum."SetInpChanCFD", enum."SetInpChanDeadtime", enum."SetBinning", enum."SetHistoOffset", enum."SetHistoLen", enum."SetStopOvl", enum."Resize", enum."EnableControls", enum."WriteStatus"] items=["Idle", "Init", "SetInpChanEnable", "SetInpChanOffset", "SetInpChanCFD", "SetInpChanTrg", "SetInpChanDeadtime", "SetSyncDivider", "SetSyncCFD", "SetSyncTrg", "SetSyncOffset", "SetBinning", "SetHistoOffset", "SetHistoLen", "SetStopOvl", "SetBitShift", "SetHistoAcqTime", "GetRates", "StartMeas", "StopMeas", "AbortMeas", "GetResolution", "GetHisto", "ReadFiFo", "WriteStatus", "Resize", "EnableControls", "DisableControls", "Error", "Exit"]
          }
        }
        n125 = property on="CFDLevel" class="DigNum (strict)"("Visible"=w201) -> ()  [unwired: 2 in, 2 out]
        n126 = property on="ZeroX" class="DigNum (strict)"("Visible"=w201) -> ()  [unwired: 2 in, 2 out]
        n127 = property on="dtcode" class="Ring (strict)"("Visible"=w201) -> ()  [unwired: 2 in, 2 out]
        n128 = property on="SyncCFDLevel" class="DigNum (strict)"("Visible"=w201) -> ()  [unwired: 2 in, 2 out]
        n129 = property on="SyncZeroX" class="DigNum (strict)"("Visible"=w201) -> ()  [unwired: 2 in, 2 out]
        n130 = local write "Binning"(w240) -> ()
        n131 = local write "HistoOffset"(w239) -> ()
        n132 = local write "HistoLength"(w237) -> ()
        n133 = local write "StopOvl."(w236) -> ()
        n134 = local write "OvlLevel"(w235) -> ()
        n135 = local write "Start"(w234) -> ()
        n136 = local write "Run continuously"(w232) -> ()
        n137 = local write "AcqTime"(w238) -> ()
        n138 = Not(x=w201) -> (.not. x?=w200:bool)
        n139 = property on="TrgLevel" class="DigNum (strict)"("Visible"=w200) -> ()  [unwired: 2 in, 2 out]
        n140 = property on="TrgEdge" class="Ring (strict)"("Visible"=w200) -> ()  [unwired: 2 in, 2 out]
        n141 = property on="SyncTrgLevel" class="DigNum (strict)"("Visible"=w200) -> ()  [unwired: 2 in, 2 out]
        n142 = property on="SyncTrgEdge" class="Ring (strict)"("Visible"=w200) -> ()  [unwired: 2 in, 2 out]
        n143 = Build Array (concatenate)(w246, w196) -> (w245:T5[])
      }
      frame "SetInpChanEnable" {
        n144 = Unbundle By Name(w281) -> ("DevIdx"=w280:i32, "Channels"=w275:T2[], "CurrentChannels"=w276:i32[])
        n145 = for {
          tunnel: w280 -> [w288]
          shift-right: [w287] -> w279
          shift-left: errorcluster {"status"=FALSE, "code"=0, "source"=""} ("error out") -> [w286]
          tunnel: w276 -> [w282] mode=indexing
          tunnel: w275 -> [w285]
          n146 = Index Array(array=w285, index=w282) -> (element=w284:T2)
          n147 = Unbundle By Name(w284) -> ("Enable"=w283:bool)
          n148 = call "TH260_SetInputChannelEnable.vi"("error in (no error)"=w286, "enable"=w283, "channel"=w282, "devidx"=w288) -> ("error out"=w287:errorcluster)  [unwired: 6 in, 1 out]
        }
      }
      frame "SetInpChanOffset" {
        n149 = Unbundle By Name(w295) -> ("DevIdx"=w294:i32, "Channels"=w289:T2[], "CurrentChannels"=w290:i32[])
        n150 = for {
          tunnel: w294 -> [w300]
          shift-right: [w297] -> w293
          shift-left: errorcluster {"status"=FALSE, "code"=0, "source"=""} ("error out") -> [w298]
          tunnel: w290 -> [w299] mode=indexing
          tunnel: w289 -> [w302]
          n151 = Index Array(array=w302, index=w299) -> (element=w301:T2)
          n152 = Unbundle By Name(w301) -> ("Offset"=w296:i32)
          n153 = call "TH260_SetInputChannelOffset.vi"("error in (no error)"=w298, "offset"=w296, "channel"=w299, "devidx"=w300) -> ("error out"=w297:errorcluster)  [unwired: 6 in, 1 out]
        }
      }
      frame "SetInpChanTrg" {
        n154 = Unbundle By Name(w309) -> ("DevIdx"=w308:i32, "Channels"=w303:T2[], "CurrentChannels"=w304:i32[])
        n155 = for {
          tunnel: w308 -> [w312]
          shift-right: [w314] -> w307
          shift-left: errorcluster {"status"=FALSE, "code"=0, "source"=""} ("error out") -> [w315]
          tunnel: w304 -> [w313] mode=indexing
          tunnel: w303 -> [w317]
          n156 = Index Array(array=w317, index=w313) -> (element=w316:T2)
          n157 = Unbundle By Name(w316) -> ("TrgLevel"=w311:i32, "TrgEdge"=w310:i32)
          n158 = call "TH260_SetInputEdgeTrg.vi"("channel"=w313, "error in (no error)"=w315, "edge"=w310, "level"=w311, "devidx"=w312) -> ("error out"=w314:errorcluster)  [unwired: 5 in, 1 out]
        }
      }
      frame "SetInpChanCFD" {
        n159 = Unbundle By Name(w324) -> ("DevIdx"=w323:i32, "Channels"=w318:T2[], "CurrentChannels"=w319:i32[])
        n160 = for {
          tunnel: w323 -> [w327]
          shift-right: [w329] -> w322
          shift-left: errorcluster {"status"=FALSE, "code"=0, "source"=""} ("error out") -> [w330]
          tunnel: w319 -> [w328] mode=indexing
          tunnel: w318 -> [w332]
          n161 = Index Array(array=w332, index=w328) -> (element=w331:T2)
          n162 = Unbundle By Name(w331) -> ("CFDLevel"=w326:i32, "ZeroX"=w325:i32)
          n163 = call "TH260_SetInputCFD.vi"("channel"=w328, "error in (no error)"=w330, "CFD ZeroCross"=w325, "CFD Level"=w326, "devidx"=w327) -> ("error out"=w329:errorcluster)  [unwired: 5 in, 1 out]
        }
      }
      frame "SetInpChanDeadtime" {
        n164 = Unbundle By Name(w339) -> ("DevIdx"=w338:i32, "Channels"=w333:T2[], "CurrentChannels"=w334:i32[])
        n165 = for {
          tunnel: w338 -> [w341]
          shift-right: [w343] -> w337
          shift-left: errorcluster {"status"=FALSE, "code"=0, "source"=""} ("error out") -> [w344]
          tunnel: w334 -> [w342] mode=indexing
          tunnel: w333 -> [w346]
          n166 = Index Array(array=w346, index=w342) -> (element=w345:T2)
          n167 = Unbundle By Name(w345) -> ("dtcode"=w340:i32)
          n168 = call "TH260_SetInputDeadTime.vi"("error in (no error)"=w344, "dtcode"=w340, "channel"=w342, "devidx"=w341) -> ("error out"=w343:errorcluster)  [unwired: 6 in, 1 out]
        }
      }
      frame "SetSyncDivider" {
        n169 = Unbundle By Name(w354) -> ("DevIdx"=w353:i32, "SyncDivider"=w349:i32)
        n170 = Power Of 2(x=w349) -> (2^x=w348:dbl)
        n171 = To Long Integer(number=w348) -> (32bit integer=w347:i32)
        n172 = call "TH260_SetSyncDiv.vi"("SyncDivider"=w347, "devidx"=w353) -> ("error out"=w351:errorcluster)  [unwired: 8 in, 1 out]
        n173 = flat-sequence {
          tunnel: w351 -> [w355]
          tunnel: [w355] -> w350
          frame #0 {
            n174 = Wait (ms)(milliseconds to wait=u32 100) -> ()  [unwired: 1 out]
          }
        }
      }
      frame "SetSyncTrg" {
        n175 = Unbundle By Name(w362) -> ("DevIdx"=w359:i32, "SyncTrgLevel"=w357:i32, "SyncTrgEdge"=w358:i32)
        n176 = call "TH260_SetSyncEdgeTrg.vi"("edge"=w358, "level"=w357, "devidx"=w359) -> ("error out"=w360:errorcluster)  [unwired: 7 in, 1 out]
      }
      frame "SetSyncCFD" {
        n177 = Unbundle By Name(w368) -> ("DevIdx"=w365:i32, "SyncCFDLevel"=w363:i32, "SyncZeroX"=w364:i32)
        n178 = call "TH260_SetSyncCFD.vi"("CFD ZeroCross"=w364, "CFD Level"=w363, "devidx"=w365) -> ("error out"=w366:errorcluster)  [unwired: 7 in, 1 out]
      }
      frame "SetSyncOffset" {
        n179 = Unbundle By Name(w373) -> ("DevIdx"=w371:i32, "SyncOffset"=w370:i32)
        n180 = call "TH260_SetSyncChannelOffset.vi"("Offset"=w370, "devidx"=w371) -> ("error out"=w372:errorcluster)  [unwired: 8 in, 1 out]
      }
      frame "SetBinning" {
        # "When binning is changed the new resolution is querried"
        n181 = Unbundle By Name(w380) -> ("DevIdx"=w378:i32, "Binning"=w377:i32)
        n182 = call "TH260_SetBinning.vi"("Binning"=w377, "devidx"=w378) -> ("error out"=w379:errorcluster)  [unwired: 8 in, 1 out]
        n183 = Build Array (concatenate)(TH260_UIThread_Cmds."GetResolution", w375) -> (w376:T5[])
      }
      frame "SetHistoOffset" {
        n184 = Unbundle By Name(w385) -> ("DevIdx"=w382:i32, "HistoOffset"=w381:i32)
        n185 = call "TH260_SetOffset.vi"("Offset"=w381, "devidx"=w382) -> ("error out"=w383:errorcluster)  [unwired: 8 in, 1 out]
      }
      frame "SetHistoLen" {
        n186 = Unbundle By Name(w388) -> ("DevIdx"=w390:i32, "HistoLen"=w389:i32)
        n187 = call "TH260_SetHistoLen.vi"("lencode"=w389, "devidx"=w390) -> ("error out"=w391:errorcluster, "actuallen"=w386:i32)  [unwired: 7 in, 1 out]
        n188 = Bundle By Name(cluster=w388, "HistoLength"=w386) -> (w387:T3)
      }
      frame "SetStopOvl" {
        n189 = Unbundle By Name(w398) -> ("DevIdx"=w395:i32, "StopOvl."=w394:bool, "OvlLevel"=w393:u32)
        n190 = call "TH260_SetStopOverflow.vi"("stopcount"=w393, "StopOnOverflow"=w394, "devidx"=w395) -> ("error out"=w396:errorcluster)  [unwired: 7 in, 1 out]
      }
      frame "GetRates" {
        n191 = Unbundle By Name(w408) -> ("Init Info.nchannels"=w406:i32, "Channels"=w399:T2[], "DevIdx"=w400:i32)
        n192 = call "TH260_GetSyncRate.vi"("devidx"=w400) -> ("error out"=w405:errorcluster, "rate"=w404:i32)  [unwired: 8 in, 1 out]
        n193 = Format Into String(format string="Sync Rate: %d cps\n", w404) -> (resulting string=→"SyncRate":string)  [unwired: 2 in, 1 out]
        n194 = for {
          N: w406 -> [_]
          tunnel: w400 -> [w415]
          tunnel: [w412] -> w402 mode=indexing
          shift-right: [w414] -> w407
          shift-left: w405 -> [w416]
          tunnel: w399 -> [w411] mode=indexing
          i -> [w413]
          n195 = Unbundle By Name(w411) -> ("Enable"=w410:bool)
          n196 = case shown="True" w410 {
            tunnel: w416 -> [w417 w422]
            tunnel: w415 -> [_ w421]
            tunnel: [w417 w420] -> w414
            tunnel: w413 -> [_ w419]
            tunnel: [_ w418] -> w412
            frame False {
            }
            frame True {
              n197 = call "TH260_GetCountRate.vi"("error in (no error)"=w422, "Channel"=w419, "devidx"=w421) -> ("error out"=w420:errorcluster, "rate"=w418:i32)  [unwired: 6 in, 1 out]
            }
          }
        }
        "CountRates" <- w402
      }
      frame "StartMeas" {
        n198 = Unbundle By Name(w430) -> ("AcqTime"=w426:i32, "DevIdx"=w427:i32)
        n199 = call "TH260_ClearHistMem.vi"("devidx"=w427) -> ("error out"=w428:errorcluster)  [unwired: 9 in, 1 out]
        n200 = call "TH260_StartMeas.vi"("error in (no error)"=w428, "Acquisition time"=w426, "devidx"=w427) -> ("error out"=w429:errorcluster)  [unwired: 7 in, 1 out]
        n201 = Build Array (concatenate)(w425, TH260_UIThread_Cmds."GetHisto") -> (w424:T5[])
      }
      frame "StopMeas" {
        n202 = Unbundle By Name(w436) -> ("Run cont."=w431:bool, "DevIdx"=w437:i32)
        n203 = call "TH260_StopMeas.vi"("devidx"=w437) -> ("error out"=w438:errorcluster)  [unwired: 9 in, 1 out]
        n204 = case shown="False" w431 {
          tunnel: w436 -> [w442 w444]
          tunnel: [w441 w444] -> w435
          tunnel: [w439 w443] -> w434
          frame False {
            w439 = T5[] [enum."GetHisto"] items=["Idle", "Init", "SetInpChanEnable", "SetInpChanOffset", "SetInpChanCFD", "SetInpChanTrg", "SetInpChanDeadtime", "SetSyncDivider", "SetSyncCFD", "SetSyncTrg", "SetSyncOffset", "SetBinning", "SetHistoOffset", "SetHistoLen", "SetStopOvl", "SetBitShift", "SetHistoAcqTime", "GetRates", "StartMeas", "StopMeas", "AbortMeas", "GetResolution", "GetHisto", "ReadFiFo", "WriteStatus", "Resize", "EnableControls", "DisableControls", "Error", "Exit"]
            w440 = FALSE ("StartMeas")
            n205 = Bundle By Name(cluster=w442, "StartMeas"=w440) -> (w441:T3)
            n206 = local write "Start"(w440) -> ()
          }
          frame True {
            w443 = T5[] [enum."GetHisto", enum."StartMeas"] items=["Idle", "Init", "SetInpChanEnable", "SetInpChanOffset", "SetInpChanCFD", "SetInpChanTrg", "SetInpChanDeadtime", "SetSyncDivider", "SetSyncCFD", "SetSyncTrg", "SetSyncOffset", "SetBinning", "SetHistoOffset", "SetHistoLen", "SetStopOvl", "SetBitShift", "SetHistoAcqTime", "GetRates", "StartMeas", "StopMeas", "AbortMeas", "GetResolution", "GetHisto", "ReadFiFo", "WriteStatus", "Resize", "EnableControls", "DisableControls", "Error", "Exit"]
          }
        }
        n207 = Build Array (concatenate)(w433, w434) -> (w432:T5[])
      }
      frame "AbortMeas" {
        w448 = T5[] [enum."GetHisto"] items=["Idle", "Init", "SetInpChanEnable", "SetInpChanOffset", "SetInpChanCFD", "SetInpChanTrg", "SetInpChanDeadtime", "SetSyncDivider", "SetSyncCFD", "SetSyncTrg", "SetSyncOffset", "SetBinning", "SetHistoOffset", "SetHistoLen", "SetStopOvl", "SetBitShift", "SetHistoAcqTime", "GetRates", "StartMeas", "StopMeas", "AbortMeas", "GetResolution", "GetHisto", "ReadFiFo", "WriteStatus", "Resize", "EnableControls", "DisableControls", "Error", "Exit"]
        w445 = FALSE ("StartMeas")
        n208 = Unbundle By Name(w450) -> ("DevIdx"=w451:i32)
        n209 = call "TH260_StopMeas.vi"("devidx"=w451) -> ("error out"=w452:errorcluster)  [unwired: 9 in, 1 out]
        n210 = Bundle By Name(cluster=w450, "StartMeas"=w445) -> (w449:T3)
        n211 = local write "Start"(w445) -> ()
        n212 = Build Array (concatenate)(w447, w448) -> (w446:T5[])
      }
      frame "GetResolution" {
        # "Resolution in ns"
        # "Gets resolution in ps"
        # "Resolution is saved in UIThread Data cluster in ns"
        n213 = Unbundle By Name(w457) -> ("DevIdx"=w459:i32)
        n214 = call "TH260_GetResolution.vi"("devidx"=w459) -> ("error out"=w458:errorcluster, "resolution"=w455:dbl)  [unwired: 8 in, 1 out]
        n215 = Divide(x=w455, y=1000.0) -> (x/y=w453:dbl)
        n216 = Bundle By Name(cluster=w457, "Resolution"=w453) -> (w456:T3)
      }
      frame "GetHisto" {
        w471 = 1  # FLAG_OVERFLOW
        # "Provides a buffer (U32-array of length 'HistoLength') for histograms."
        n217 = Unbundle By Name(w486) -> ("Resolution"=w483:dbl, "Init Info.nchannels"=w463:i32, "Channels"=w464:T2[], "DevIdx"=w485:i32, "HistoLength"=w484:i32)
        n218 = call "TH260_AllocateHistoBuffer.vi"("HistoLength"=w484) -> ("Buffer"=w477:u32[])  [unwired: 10 in]
        n219 = property class="VI"() -> ("Panel"=w462:refnum<vi>)  [unwired: 2 in, 2 out]
        n220 = for {
          N: w463 -> [_]
          tunnel: w485 -> [w500]
          tunnel: [w497] -> w474 mode=indexing
          tunnel: w477 -> [w498]
          shift-right: [w499] -> w473
          shift-left: errorcluster {"status"=FALSE, "code"=0, "source"=""} ("error IO") -> [w491]
          shift-right: [w492] -> w466
          shift-left: "Total Counts:\t\t" -> [w490]
          tunnel: w464 -> [w489] mode=indexing
          i -> [w496]
          n221 = Unbundle By Name(w489) -> ("Enable"=w488:bool)
          n222 = case shown="True" w488 {
            tunnel: w500 -> [_ w509]
            tunnel: [w501 w508] -> w499
            tunnel: w498 -> [w502 w507]
            tunnel: [w502 w506] -> w497
            tunnel: w496 -> [_ w505]
            tunnel: w491 -> [w501 w504]
            frame False {
            }
            frame True {
              n223 = call "TH260_GetHistogram.vi"("devidx"=w509, "Buffer"=w507, "clear"=FALSE, "error in (no error)"=w504, "channel"=w505) -> ("Histogram"=w506:u32[], "error out"=w508:errorcluster)  [unwired: 3 in, 1 out]
            }
          }
          n224 = Add Array Elements(numeric array=w497) -> (sum=w493:u32)
          n225 = Increment(x=w496) -> (x+1=w494:i32)
          n226 = Format Into String(format string="Ch.%2d: %d cnts.\t\t", initial string=w490, w494, w493) -> (resulting string=w492:string)  [unwired: 1 in, 1 out]
        }
        n227 = property class="Pnl"(reference=w462, "DeferPanUpdts"=FALSE ("Defer Panel Updates")) -> ()  [unwired: 1 in, 2 out]
        n228 = call "CalcRate.vi"("Refresh(ms)"=u32 500) -> ("Rate / Hz"=w481:dbl)  [unwired: 8 in, 2 out]
        n229 = Format Into String(format string="Readout Rate: %.1f Hz\\t\\t", w481) -> (resulting string=w479:string)  [unwired: 2 in, 1 out]
        n230 = Concatenate Strings(w479, w466) -> (w478:string)
        n231 = Bundle(0.0, "Resolution"=w483, "Histogram"=w474) -> (→"HistoGraph":T1)  [unwired: 1 in]
        n232 = local write "Status"(w478) -> ()
        n233 = call "TH260_GetFlags.vi"("error in (no error)"=w473) -> ("error out"=w482:errorcluster, "flags"=w470:i32)  [unwired: 8 in, 1 out]
        n234 = And(x=w471, y=w470) -> (x .and. y?=w472:i32)
        n235 = Not Equal To 0?(x=w472) -> (x != 0?=→"OverFlow":bool)
      }
      frame "WriteStatus" {
        n236 = Unbundle By Name(w511) -> ("Status"=→"Status":string)
      }
      frame "Resize" {
        n237 = property on="Pane 3" class="Pane"() -> ("Width"=w518:u32)  [unwired: 2 in, 2 out]
        n238 = Subtract(x=w518, y=i16 100 ("b")) -> (x-y=w524:u32)
        n239 = Unbundle By Name(w513) -> ("Init Info.nchannels"=w521:i32)
        n240 = Quotient & Remainder(x=w524, y=i16 99 ("m")) -> (floor(x/y)=w523:u32)  [unwired: 1 out]
        n241 = In Range and Coerce(upper limit=w521, x=w523, lower limit=4) -> (coerced(x)=w522:u32)  [unwired: 1 out]
        n242 = Equal?(x=w521, y=w522) -> (x = y?=w520:bool)
        n243 = Not(x=w520) -> (.not. x?=w519:bool)
        n244 = property on="Channels" class="Arr (strict)"("HorizScroll"=w519, "Number of Columns"=w522, "Index Values"=u32[] [0]) -> ()  [unwired: 2 in, 2 out]
      }
      frame "EnableControls" {
        n245 = property class="VI"() -> ("Panel"=w529:refnum<vi>)  [unwired: 2 in, 2 out]
        n246 = property class="Pnl"(reference=w529) -> ("Controls[]"=w528:refnum<vi>[])  [unwired: 1 in, 2 out]
        n247 = property class="Pnl"(reference=w529) -> ("Decos[]"=w530:refnum<vi>[])  [unwired: 1 in, 2 out]
        n248 = for {
          tunnel: w530 -> [w534] mode=indexing
          tunnel: TRUE -> [w533]
          n249 = property class="Decor"(reference=w534, "Visible"=w533) -> ()  [unwired: 1 in, 2 out]
        }
        n250 = for {
          tunnel: w528 -> [w537] mode=indexing
          tunnel: T6."Enabled" ("Disabled") -> [w536]
          tunnel: [w535] -> _
          n251 = property class="Ctl"(reference=w537, "DisabledEnum"=w536) -> (error out=w535:errorcluster)  [unwired: 1 in, 1 out]
        }
      }
      frame "DisableControls" {
        n252 = property class="VI"() -> ("Panel"=w541:refnum<vi>)  [unwired: 2 in, 2 out]
        n253 = property class="Pnl"(reference=w541) -> ("Controls[]"=w540:refnum<vi>[])  [unwired: 1 in, 2 out]
        n254 = property class="Pnl"(reference=w541) -> ("Decos[]"=w542:refnum<vi>[])  [unwired: 1 in, 2 out]
        n255 = for {
          tunnel: w542 -> [w546] mode=indexing
          tunnel: FALSE -> [w545]
          n256 = property class="Decor"(reference=w546, "Visible"=w545) -> ()  [unwired: 1 in, 2 out]
        }
        n257 = for {
          tunnel: w540 -> [w549] mode=indexing
          tunnel: T6."Disabled and Grayed Out" ("Disabled") -> [w548]
          tunnel: [w547] -> _
          n258 = property class="Ctl"(reference=w549, "DisabledEnum"=w548) -> (error out=w547:errorcluster)  [unwired: 1 in, 1 out]
        }
      }
      frame "Error" {
        w550 = T5[] [enum."Exit"] items=["Idle", "Init", "SetInpChanEnable", "SetInpChanOffset", "SetInpChanCFD", "SetInpChanTrg", "SetInpChanDeadtime", "SetSyncDivider", "SetSyncCFD", "SetSyncTrg", "SetSyncOffset", "SetBinning", "SetHistoOffset", "SetHistoLen", "SetStopOvl", "SetBitShift", "SetHistoAcqTime", "GetRates", "StartMeas", "StopMeas", "AbortMeas", "GetResolution", "GetHisto", "ReadFiFo", "WriteStatus", "Resize", "EnableControls", "DisableControls", "Error", "Exit"]
        w553 = T9 1 items=["no dialog", "OK message", "continue or stop message", "OK message + warnings", "continue/stop + warnings"] ("type of dialog (OK msg:1)")
        # "Error case: If an error occures the user is informed and the programm terminates. Add your own code to handle error events (e.g. exception lists, etc.)"
        n259 = call <vilib>:"Simple Error Handler.vi"("type of dialog (OK msg:1)"=w553, "error in (no error)"=w552) -> ()  [unwired: 3 in, 5 out]
      }
      frame "Exit" {
        n260 = Unbundle By Name(w557) -> ("DevIdx"=w556:i32)
        n261 = call "TH260_CloseDevice.vi"("devidx"=w556) -> ("error out"=w555:errorcluster)  [unwired: 9 in, 1 out]
      }
    }
    n262 = call "TH260_EnQError.vi"("error in (no error)"=w8, "Cmds_in"=w6) -> ("error out"=w7:errorcluster, "Cmds_out"=w5:T5[])  [unwired: 8 in]
  }
